vi "Trick101Register.vi"(6 "channel":i32, 7 "adder":i32, 8 "error in":errorcluster, 11 "connection ID":refnum<k5>) -> (0 "error out":errorcluster, 3 "connection ID out":refnum<k5>)   [LabVIEW 2012]
panel:
  out "data out serial":string="0_2-63@36\r\n"
  out "element":i32
  in  "Register Value":i32[](array[numeric])=[1816, 1840, 1832, 1848, 1, 1, 1]
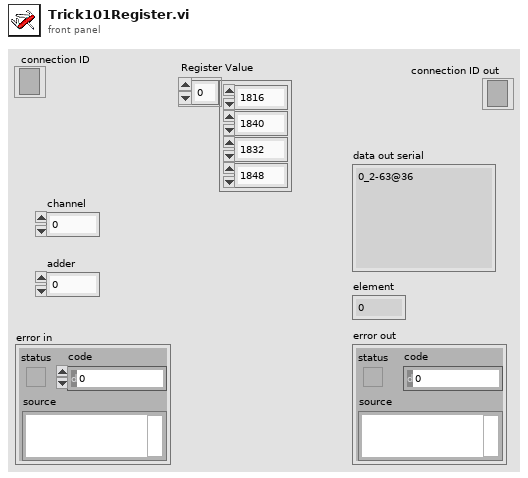
[diagram p1: front panel]
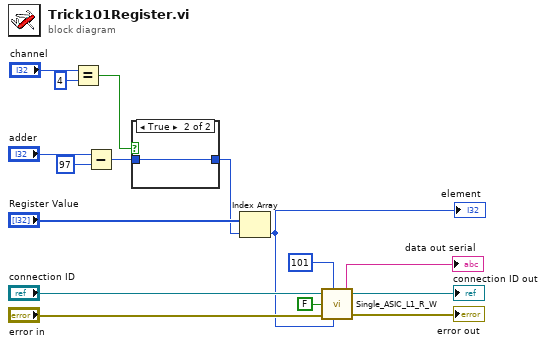
[diagram p0: block diagram]
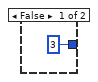
[diagram p2: hidden frame]
diagram:
  n1 = Equal?(x="channel", y=4) -> (x = y?=w1:bool)
  n2 = Subtract(x="adder", y=97) -> (x-y=w2:i32)
  n3 = case shown="True" w1 {
    tunnel: [3 w18] -> w3
    tunnel: w2 -> [_ w18]
    frame False {
    }
    frame True {
    }
  }
  n4 = Index Array(array="Register Value", index=w3) -> (element=w9:i32)
  "element" <- w9
  n5 = call "Single_ASIC_L1_R_W.vi"("connection ID"="connection ID", "Register or channel"=101, "RD/#WR"=FALSE, "error in (no error)"="error in", "Data"=w9) -> ("data out serial"=→"data out serial":string, "connection ID out"=→"connection ID out":refnum<k5>, "error out"=→"error out":errorcluster)  [unwired: 1 in, 1 out]
